vi "Tosca-Save AI Plot Properties.vi"(0 "plot":T1, 11 "error in (no error)":errorcluster) -> ()   [LabVIEW 2020]
uses:
  Typedefs/Tosca-AI Plot Properties.ctl
panel:
  out "Error Out":errorcluster
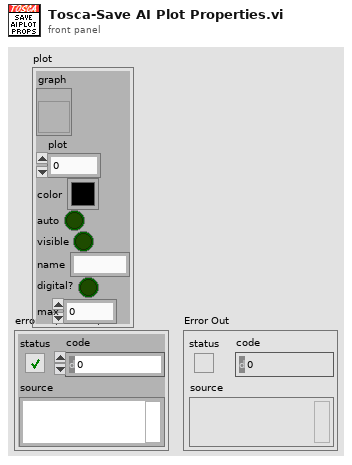
[diagram p1: front panel]
types:
  T1 = typedef "Tosca-AI Plot Properties.ctl" = cluster{"graph":refnum<vi>, "plot":i32, "color":u32, "auto":bool, "visible":bool, "name":string, "digital?":bool, "max":dbl}
  T2 = cluster{"color":u32, "visible":bool, "auto":bool, "max":dbl}
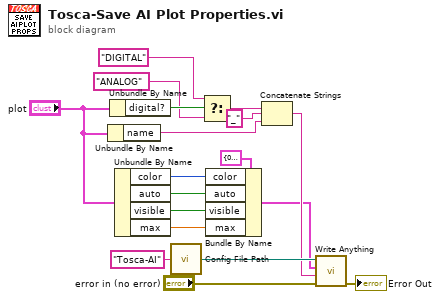
[diagram p0: block diagram]
diagram:
  n1 = Unbundle By Name("plot") -> ("name"=w9:string)
  n2 = Unbundle By Name("plot") -> ("digital?"=w13:bool)
  n3 = Unbundle By Name("plot") -> ("color"=w5:u32, "auto"=w4:bool, "visible"=w3:bool, "max"=w1:dbl)
  n4 = call "Config File Path.vi"("AppName"="Tosca-AI") -> ("Default config file name"=w17:path)
  n5 = Select(t="DIGITAL", s=w13, f="ANALOG") -> (s? t:f=w10:string)
  n6 = Bundle By Name(cluster=T2 {"color"=0, "visible"=FALSE, "auto"=FALSE, "max"=0.0}, "color"=w5, "auto"=w4, "visible"=w3, "max"=w1) -> (w7:T2)
  n7 = Concatenate Strings(w10, "_" ("string"), w9) -> (w14:string)
  n8 = call "Write Anything.vi"("Error In"="error in (no error)", "Section Name (Name of \"Anything\")"=w14, "Anything"=w7, "Path (dialog)"=w17) -> ("Error Out"=→"Error Out":errorcluster)  [unwired: 6 in, 1 out]
